vi "Clean form.vi"(11 "html in":string="sdfsfsse") -> (0 "after hyperlink":string, 1 "text":string, 2 "link":string, 3 "before hyperlink":string, 4 "Success?":bool)   [LabVIEW 2020]
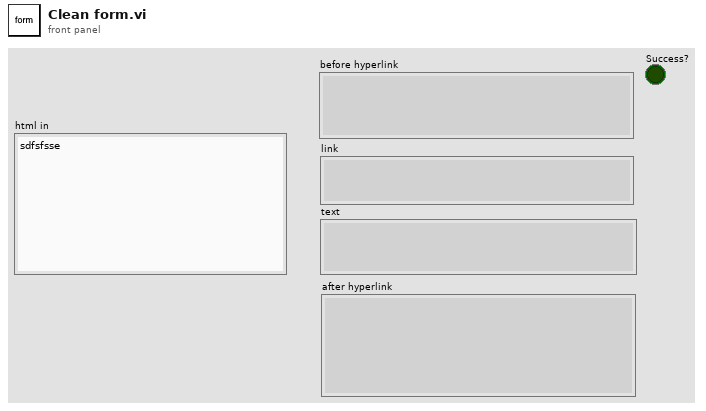
[diagram p1: front panel]
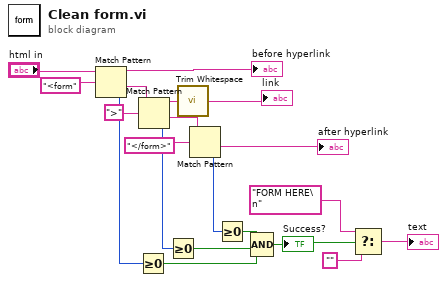
[diagram p0: block diagram]
diagram:
  n1 = Match Pattern(string="html in", regular expression="<form" ("format string")) -> (before substring=→"before hyperlink":string, after substring=w18:string, offset past match=w10:i32)  [unwired: 1 in, 1 out]
  n2 = Greater Or Equal To 0?(x=w10) -> (x >= 0?=w5:bool)
  n3 = Match Pattern(string=w18, regular expression=">" ("format string")) -> (before substring=w14:string, after substring=w15:string, offset past match=w9:i32)  [unwired: 1 in, 1 out]
  n4 = Greater Or Equal To 0?(x=w9) -> (x >= 0?=w6:bool)
  n5 = call <vilib>:"Trim Whitespace.vi"("string"=w14) -> ("trimmed string"=→"link":string)  [unwired: 1 in]
  n6 = Match Pattern(string=w15, regular expression="</form>" ("format string")) -> (after substring=→"after hyperlink":string, offset past match=w8:i32)  [unwired: 1 in, 2 out]
  n7 = Greater Or Equal To 0?(x=w8) -> (x >= 0?=w7:bool)
  n8 = Compound Arithmetic op=AND(w7, w6, w5) -> (w4:bool)
  "Success?" <- w4
  n9 = Select(t="FORM HERE\n" ("text"), s=w4, f="") -> (s? t:f=→"text":string)
